vi "Create.vi"(7 "Direction":enum16{"North", "East", "South", "West"}(ring), 8 "error in (no error)":errorcluster, 9 "Col":i32, 10 "Row":i32) -> (0 "error out":errorcluster, 3 "Beam":refnum<class "Beam.lvclass">)   [LabVIEW 2021, in "Beam.lvclass"]
uses:
  Beam.lvclass
  Beam.lvclass/Beam.ctl
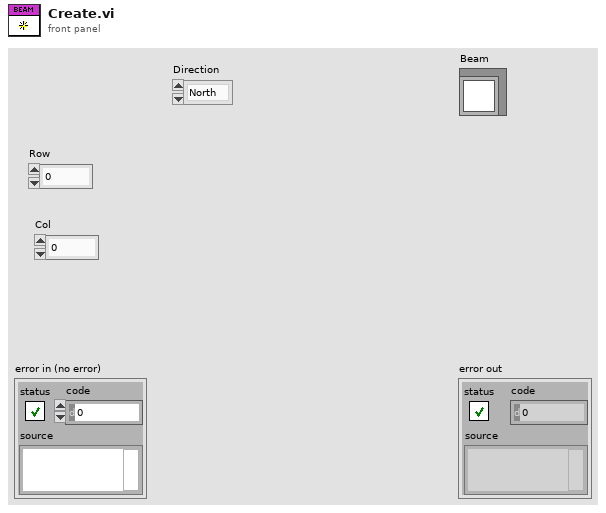
[diagram p1: front panel]
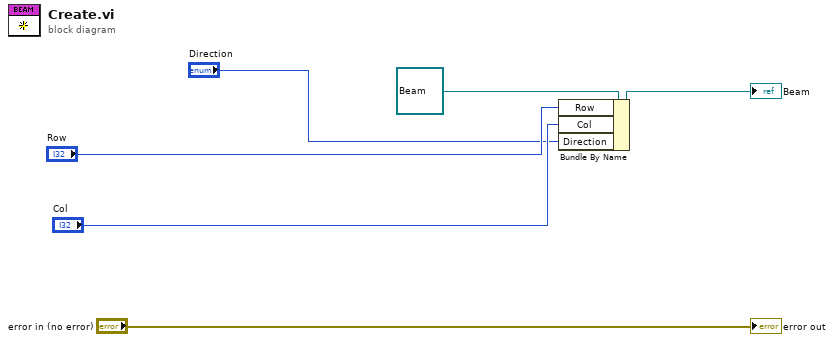
[diagram p0: block diagram]
diagram:
  n1 = Bundle By Name(cluster=refnum<class "Beam.lvclass"> refnum ("Beam"), "Row"="Row", "Col"="Col", "Direction"="Direction") -> (→"Beam":refnum<class "Beam.lvclass">)
  "error out" <- "error in (no error)"
